vi "JTAG Close.vi"(8 "error in (no error)":errorcluster, 11 "Power Target Device":bool) -> (0 "error out":errorcluster)   [LabVIEW 2010]
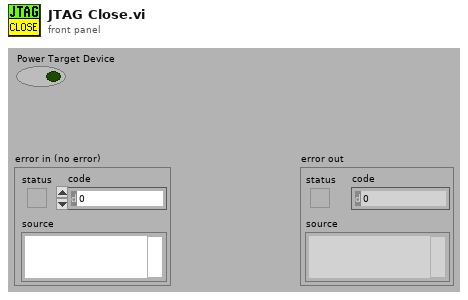
[diagram p1: front panel]
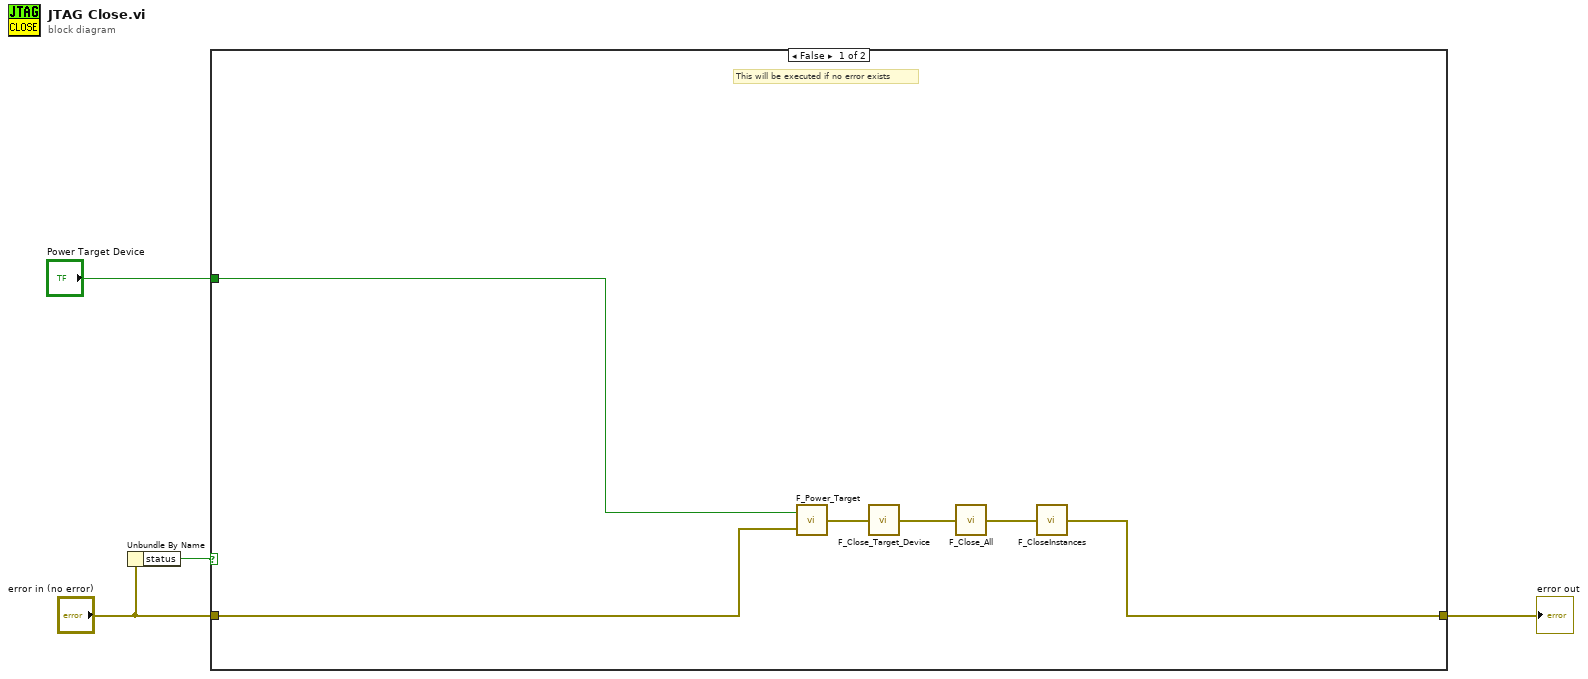
[diagram p0: block diagram]
diagram:
  n1 = Unbundle By Name("error in (no error)") -> ("status"=w3:bool)
  n2 = case shown="False" w3 {
    tunnel: [w9 w11] -> w4
    tunnel: "error in (no error)" -> [w10 w11]
    tunnel: "Power Target Device" -> [w8 _]
    frame False {
      # "This will be executed if no error exists"
      n3 = call "F_Power_Target.vi"("error in (no error)"=w10, "Power Target Device"=w8) -> ("error out"=w5:errorcluster)  [unwired: 1 in]
      n4 = call "F_Close_Target_Device.vi"("error in (no error)"=w5) -> ("error out"=w6:errorcluster)
      n5 = call "F_Close_All.vi"("error in (no error)"=w6) -> ("error out"=w7:errorcluster)
      n6 = call "F_CloseInstances.vi"("error in (no error)"=w7) -> ("error out"=w9:errorcluster)
    }
    frame True {
      # "Error exists, skip all functions"
    }
  }
  "error out" <- w4
